vi "Lock Publication.vi"(4 "Return Error Transport":refnum<class "ITransport.lvclass">, 6 "Publisher ID":string, 7 "PublicationPolicy":refnum<class "IPublicationPolicy.lvclass">, 8 "error in (no error)":errorcluster, 9 "Datum Type":variant, 10 "Datum Name":string, 11 "Mediator In":refnum<class "BusMediator.lvclass">) -> (0 "error out":errorcluster, 3 "Mediator Out":refnum<class "BusMediator.lvclass">)   [LabVIEW 2017, in "BusMediator.lvclass"]
doc: "<License>\nCopyright © 2017 Composed Systems, LLC | All rights reserved\nwww.composed.io\n\nAuthor: Ethan Stern <ethan.stern@composed.io>\n\nThis software is provided \"AS IS\" WITHOUT WARRANTIES, either express or implied, AND IS FOR EDUCATIONAL PURPOSES ONLY.\n</License>"
uses:
  BusMediator.lvclass
  <vilib>/Composed/GPM Packages/mva-framework/Source/Framework/IMediator/IPublicationPolicy/IPublicationPolicy.lvclass
  <vilib>/Composed/GPM Packages/transport/Source/ITransport/ITransport.lvclass
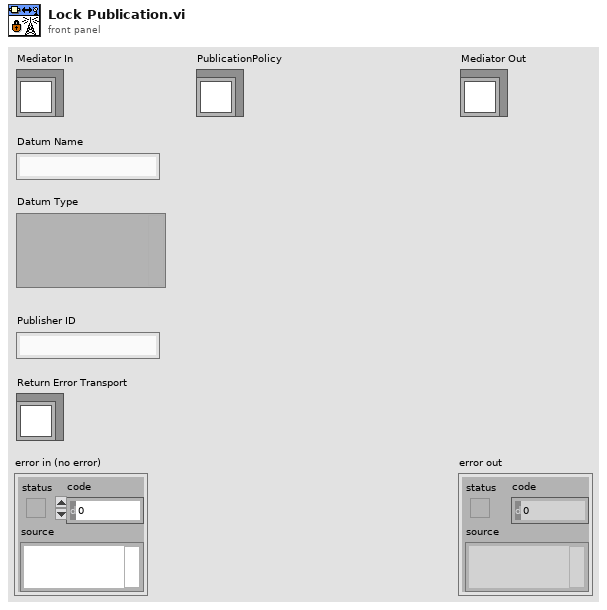
[diagram p1: front panel]
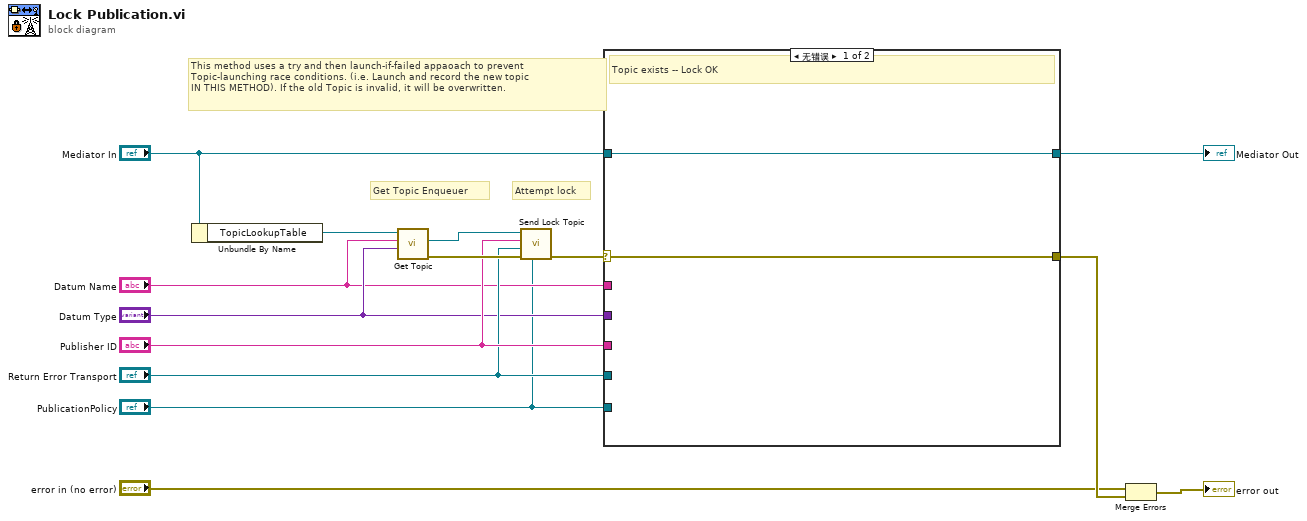
[diagram p0: block diagram]
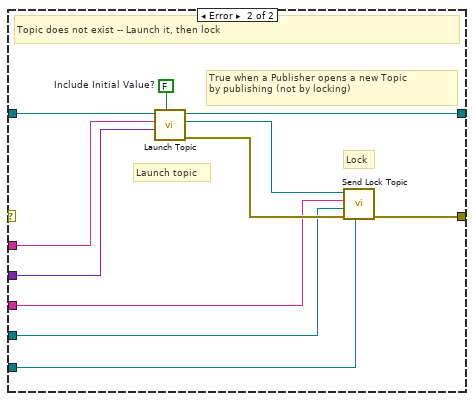
[diagram p2: hidden frame]
diagram:
  # "This method uses a try and then launch-if-failed appaoach to prevent\nTopic-launching race conditions. (i.e. Launch and record the new topic\nIN THIS METHOD). If the old Topic is invalid, it will be overwritten."
  # "Attempt lock"
  # "Get Topic Enqueuer"
  n1 = Unbundle By Name("Mediator In") -> ("TopicLookupTable"=w14:refnum<data-value>)
  n2 = call "Get Topic.vi"("Topic Type"="Datum Type", "Topic Name"="Datum Name", "TopicLookupTable"=w14) -> ("error out"=w12:errorcluster, "Topic Enqueuer"=w13:refnum<class "Message Enqueuer.lvclass">)  [unwired: 6 in, 1 out]
  n3 = call "Send Lock Topic.vi"("PublicationPolicy"="PublicationPolicy", "error in (no error)"=w12, "Return Error Transport"="Return Error Transport", "Publisher ID"="Publisher ID", "Message Enqueuer"=w13) -> ("error out"=w8:errorcluster)  [unwired: 5 in, 1 out]
  n4 = case shown="无错误" w8 {
    selector: w8 -> [w15 _]
    tunnel: "Mediator In" -> [w16 w27]
    tunnel: [w16 w25] -> w6
    tunnel: "Datum Name" -> [_ w23]
    tunnel: "Datum Type" -> [_ w22]
    tunnel: [w15 w26] -> w11
    tunnel: "Publisher ID" -> [_ w18]
    tunnel: "Return Error Transport" -> [_ w19]
    tunnel: "PublicationPolicy" -> [_ w17]
    frame No Error {
      # "Topic exists -- Lock OK"
    }
    frame Error {
      w20 = FALSE  # Include Initial Value?
      # "True when a Publisher opens a new Topic\nby publishing (not by locking)"
      # "Launch topic"
      # "Lock"
      # "Topic does not exist -- Launch it, then lock"
      n5 = call "Launch Topic.vi"("Include Initial Value? (F)"=w20, "Type"=w22, "Datum Name"=w23, "Mediator in"=w27) -> ("error out"=w21:errorcluster, "New Topic Enqueuer"=w24:refnum<class "Message Enqueuer.lvclass">, "Mediator out"=w25:refnum<class "BusMediator.lvclass">)  [unwired: 5 in]
      n6 = call "Send Lock Topic.vi"("PublicationPolicy"=w17, "error in (no error)"=w21, "Return Error Transport"=w19, "Publisher ID"=w18, "Message Enqueuer"=w24) -> ("error out"=w26:errorcluster)  [unwired: 5 in, 1 out]
    }
  }
  "Mediator Out" <- w6
  n7 = Merge Errors("error in (no error)", w11) -> (→"error out":errorcluster)
